vi "Write List of Functions.vi"(8 "error in (no error)":errorcluster, 10 "List of Functions":string[](array[string]), 11 "List of Functions Message in":refnum<class "List of Functions Message.lvclass">) -> (0 "error out":errorcluster, 3 "List of Functions Message out":refnum<class "List of Functions Message.lvclass">)   [LabVIEW 2016, in "Controller UI.lvlib" / "List of Functions Message.lvclass"]
uses:
  <userlib>/Common Components/Controller UI/Messages/List of Functions Message/List of Functions Message.lvclass
  <userlib>/Common Components/Controller UI/Messages/List of Functions Message/List of Functions Message.lvclass/List of Functions Message.ctl
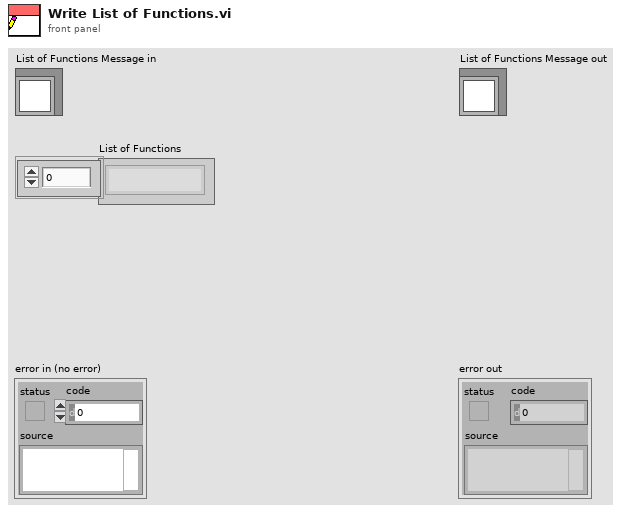
[diagram p1: front panel]
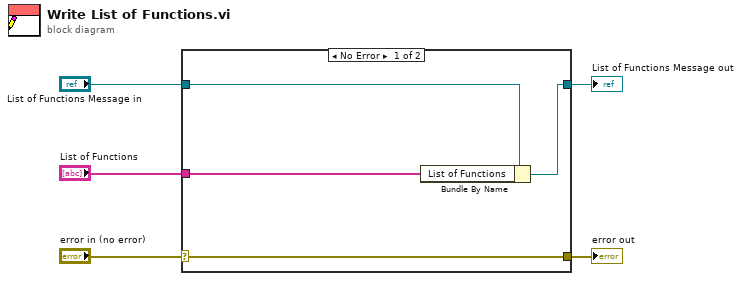
[diagram p0: block diagram]
diagram:
  n1 = case shown="No Error" "error in (no error)" {
    selector: "error in (no error)" -> [w9 w10]
    tunnel: [w9 w10] -> w4
    tunnel: [w7 w11] -> w2
    tunnel: "List of Functions Message in" -> [w8 w11]
    tunnel: "List of Functions" -> [w6 _]
    frame No Error {
      n2 = Bundle By Name(cluster=w8, "List of Functions"=w6) -> (w7:refnum<class "List of Functions Message.lvclass">)
    }
    frame Error {
    }
  }
  "error out" <- w4
  "List of Functions Message out" <- w2
